vi "Do_pulse_train.vi"(6 "error in":errorcluster, 7 "Parameters":T3 {"Acquisition parameters"."Pixels to integrate" min=1 step=1; "Acquisition parameters"."Sample rate" min=10.0 max=25000.0; "Acquisition parameters"."Clock source" items=["OnboardClock", "ExternalClock", "NoClock"]; "Stimulation parameters"."Stim onset" min=0.0 max=100.0 step=1.0; "Stimulation parameters"."Total duration" min=1.0 max=100.0 step=1.0; "Stimulation parameters"."Stim frequency" min=1.0 max=40.0 step=1.0}, 8 "Time":dbl, 9 "Stim task in":refnum<k24>) -> (0 "error out":errorcluster, 3 "stim task out":refnum<k24>)   [LabVIEW 2010]
uses:
  C:/Program Files (x86)/National Instruments/LabVIEW 2010/vi.lib/ULx/ULx_LV.dll
  Program Files (x86)/National Instruments/LabVIEW 2010/vi.lib/ULx/ULx_LV.dll
  typedefs/stimulation_parameters.ctl
  typedefs/acquisition_parameters_cluster.ctl
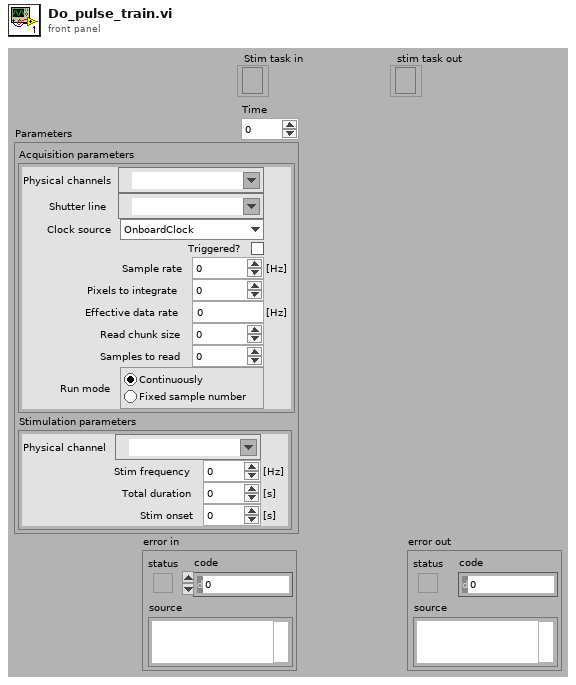
[diagram p1: front panel]
types:
  T1 = typedef "acquisition_parameters_cluster.ctl" = cluster{"Physical channels":refnum<k21>, "Shutter line":refnum<k21>, "Clock source":i32, "Triggered?":bool, "Sample rate":dbl, "Pixels to integrate":i32, "Effective data rate":dbl, "Read chunk size":i32, "Samples to read":i32, "Run mode":enum32{"Continuously", "Fixed sample number"}}
  T2 = typedef "stimulation_parameters.ctl" = cluster{"Physical channel":refnum<k21>, "Stim frequency":dbl, "Total duration":dbl, "Stim onset":dbl}
  T3 = cluster{"Acquisition parameters":T1, "Stimulation parameters":T2}
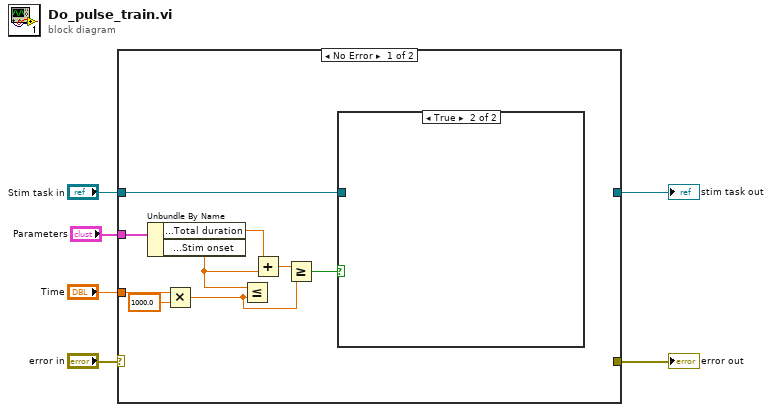
[diagram p0: block diagram]
diagram:
  n1 = case shown="No Error" "error in" {
    selector: "error in" -> [_ w17]
    tunnel: [_ w17] -> w6
    tunnel: [_ w16] -> w5
    tunnel: "Stim task in" -> [w12 w16]
    tunnel: "Time" -> [w14 _]
    tunnel: "Parameters" -> [w15 _]
    frame No Error {
      n2 = Unbundle By Name(w15) -> ("Stimulation parameters.Total duration"=w11:dbl, "Stimulation parameters.Stim onset"=w10:dbl)
      n3 = Multiply(x=w14, y=1000.0) -> (x*y=w7:dbl)
      n4 = Less Or Equal?(x=w10, y=w7) -> ()  [unwired: 1 out]
      n5 = Add(x=w11, y=w10) -> (x+y=w9:dbl)
      n6 = Greater Or Equal?(x=w9, y=w7) -> (x >= y?=w8:bool)
      n7 = case shown="True" w8 {
        tunnel: w12 -> [_ _]
        frame False {
        }
        frame True {
        }
      }
    }
    frame Error {
    }
  }
  "error out" <- w6
  "stim task out" <- w5
